vi "RF_TxParaConf.vi"(8 "error in":errorcluster, 10 "硬件\n参数\n设置":T2, 11 "VISA IN":T1) -> (0 "error OUT":errorcluster)   [LabVIEW 2015]
uses:
  <vilib>/Instr/_visa.llb/VISA Flush IO Buffer Mask.ctl
  <vilib>/Instr/_visa.llb/VISA Configure Serial Port (Instr).vi
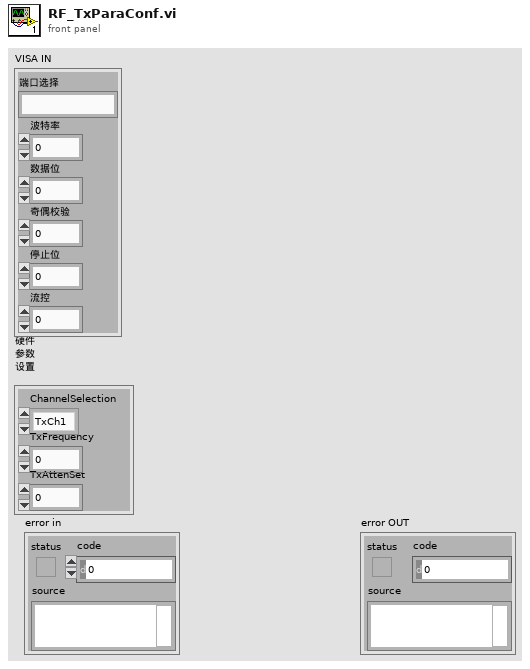
[diagram p1: front panel]
types:
  T1 = cluster{"端口选择":string, "波特率":u32, "数据位":u16, "奇偶校验":u16, "停止位":u16, "流控":u16}
  T2 = cluster{"ChannelSelection":enum16{"TxCh1", "TxCh2"}, "TxFrequency":u32, "TxAttenSet":u8}
  T3 = typedef "VISA Flush IO Buffer Mask.ctl" = u16
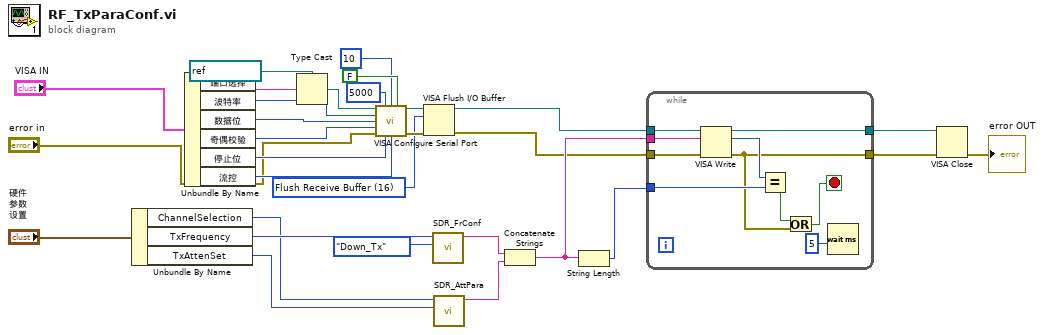
[diagram p0: block diagram]
diagram:
  w12 = T3 16 items=["Flush Receive Buffer"=16, "Write Transmit Buffer to Device"=32, "Flush Receive Buffer (No I/O)"=64, "Flush Transmit Buffer"=128] ("Mask")
  n1 = Unbundle By Name("硬件\n参数\n设置") -> ("ChannelSelection"=w28:enum16{"TxCh1", "TxCh2"}, "TxFrequency"=w29:u32, "TxAttenSet"=w27:u8)
  n2 = Unbundle By Name("VISA IN") -> ("端口选择"=w10:string, "波特率"=w16:u32, "数据位"=w20:u16, "奇偶校验"=w19:u16, "停止位"=w18:u16, "流控"=w17:u16)
  n3 = Type Cast(type=refnum<visa-resource-name> "COM15" ("VISA resource name"), x=w10) -> (*(type *) &x=w8:refnum<visa-resource-name>)
  n4 = call-poly "VISA Configure Serial Port"("VISA resource name"=w8, "timeout (10sec)"=u32 5000, "termination char\n(0xA = '\\n' = LF)"=u8 10 ("termination char\n(0xA = '\\n' = LF)"), "Enable Termination\nChar (T)"=FALSE ("Enable Termination Char (T)"), "baud rate (9600)"=w16, "data bits (8)"=w20, "parity (0:none)"=w19, "error in (no error)"="error in", "stop bits (10: 1 bit)"=w18, "flow control (0:none)"=w17) -> ("VISA resource name out"=w14:refnum<visa-resource-name>, "error out"=w13:errorcluster)  [unwired: 4 out]
  n5 = VISA Flush I/O Buffer(VISA resource name=w14, mask (16)=w12, error in (no error)=w13) -> (VISA resource name out=w6:refnum<visa-resource-name>, error out=w7:errorcluster)
  n6 = call "SDR_FrConf.vi"("UpDw_Ch"=enum16{"Up_Rx", "Down_Tx"}."Down_Tx", "RxFrequency"=w29) -> ("string"=w25:string)  [unwired: 9 in]
  n7 = call "SDR_AttPara.vi"("TX1衰减"=w27, "ChannelSelection"=w28) -> ("AttPara"=w24:string)  [unwired: 9 in]
  n8 = Concatenate Strings(w25, w24) -> (w23:string)
  n9 = String Length(string=w23) -> (length=w22:i32)
  n10 = while {
    tunnel: w6 -> [w40]
    tunnel: [w39] -> w2
    tunnel: w23 -> [w38]
    tunnel: w22 -> [w37]
    tunnel: w7 -> [w35]
    tunnel: [w32] -> w1
    stop <- w33 stop-if-true
    n11 = VISA Write(VISA resource name=w40, write buffer=w38, error in (no error)=w35) -> (VISA resource name out=w39:refnum<visa-resource-name>, return count=w36:u32, error out=w32:errorcluster)
    n12 = Equal?(x=w36, y=w37) -> (x = y?=w34:bool)
    n13 = Or(x=w34, y=w32) -> (x .or. y?=w33:bool)
    n14 = Wait (ms)(milliseconds to wait=u32 5) -> ()  [unwired: 1 out]
  }
  n15 = VISA Close(VISA resource name=w2, error in (no error)=w1) -> (error out=→"error OUT":errorcluster)
